vi "簇到数组.vi"() -> ()   [LabVIEW 2018]
panel:
  out "数组 2":string[](array[string])
  out "数组":dbl[](array[numeric])
  in  "簇 2":cluster{"字符串":string, "字符串 2":string}
  in  "簇":cluster{"数值":dbl, "数值 2":dbl, "数值 3":dbl}
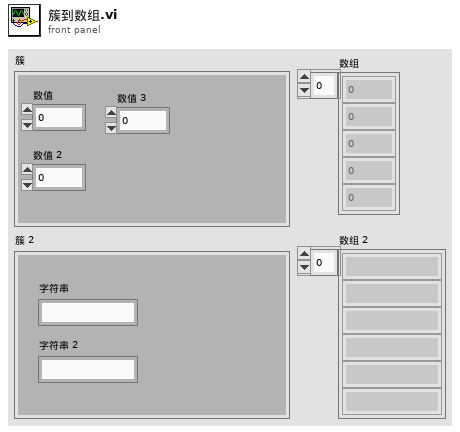
[diagram p1: front panel]
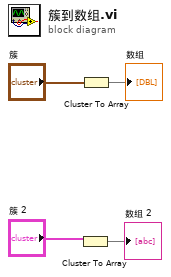
[diagram p0: block diagram]
diagram:
  n1 = Cluster To Array(cluster="簇 2") -> (array=→"数组 2":string[])
  n2 = Cluster To Array(cluster="簇") -> (array=→"数组":dbl[])
